vi "CloseDataLogFile.vi"(1 "Data Log File Refnum":refnum<k1>) -> (0 "error out":errorcluster)   [LabVIEW 2012]
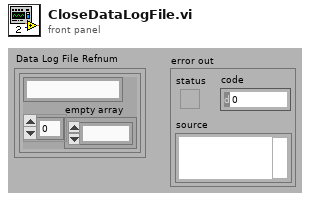
[diagram p1: front panel]
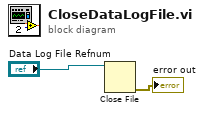
[diagram p0: block diagram]
diagram:
  n1 = Close File(refnum="Data Log File Refnum") -> (error out=→"error out":errorcluster)  [unwired: 1 in, 1 out]
